vi "Execute.vi"(7 "Data":refnum<class "Abstract.lvclass">=refnum, 8 "Error In":errorcluster, 11 "Input":string) -> (0 "Error Out":errorcluster, 3 "Output":string)   [LabVIEW 2018, in "Toolkit.lvlib"]
uses:
  Toolkit.lvlib
  Readers/String/String.lvclass
  Parser/Parser.lvclass
  Low-Level/Support/Render to String.vi
  D:/Users/cfield/Code/Field R&D Services/Mustache/trunk/src/Toolkit/Readers/Abstract/Abstract.lvclass
  Tokens/Abstract/Abstract.lvclass
  Data/Abstract/Abstract.lvclass
  Data/Map/Map.lvclass
  Data/String/String.lvclass
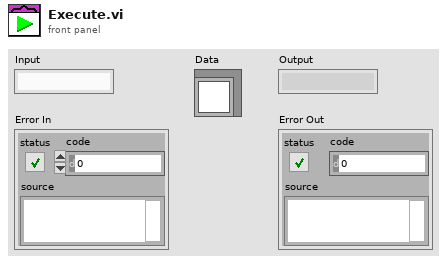
[diagram p1: front panel]
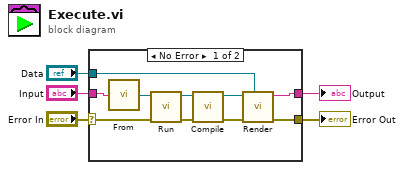
[diagram p0: block diagram]
diagram:
  n1 = case shown="No Error" "Error In" {
    selector: "Error In" -> [w6 w16]
    tunnel: [w10 w16] -> w5
    tunnel: "Input" -> [w9 w17]
    tunnel: [w8 w17] -> w3
    tunnel: "Data" -> [w7 _]
    frame No Error {
      n2 = call "From.vi"("String"=w9) -> ("String"=w15:refnum<class "String.lvclass">)
      n3 = call "Run.vi"("Error In"=w6, "Parser In"=w15) -> ("Error Out"=w12:errorcluster, "Parser Out"=w14:refnum<class "Parser.lvclass">)  [unwired: 7 in, 1 out]
      n4 = call "Compile.vi"("Error In"=w12, "Tokens"=w14) -> ("Error Out"=w11:errorcluster, "Template"=w13:refnum<class "Template.lvclass">)  [unwired: 8 in]
      n5 = call-poly "Render.vi"("Data"=w7, "Error In"=w11, "Template"=w13) -> ("Error Out"=w10:errorcluster, "Output"=w8:string)  [unwired: 7 in]
    }
    frame Error {
    }
  }
  "Error Out" <- w5
  "Output" <- w3
